vi "Checkbarcode.vi"(10 "String In":string="123456789\u0003") -> (2 "Complete":bool)   [LabVIEW 2014]
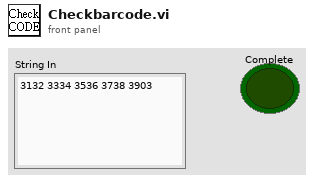
[diagram p1: front panel]
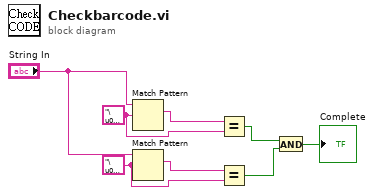
[diagram p0: block diagram]
diagram:
  w6 = "\u0003" ("regular expression")
  w1 = "\u0002" ("regular expression")
  n1 = Match Pattern(string="String In", regular expression=w1) -> (match substring=w8:string)  [unwired: 1 in, 3 out]
  n2 = Match Pattern(string="String In", regular expression=w6) -> (match substring=w7:string)  [unwired: 1 in, 3 out]
  n3 = Equal?(x=w8, y=w1) -> (x = y?=w5:bool)
  n4 = Equal?(x=w7, y=w6) -> (x = y?=w4:bool)
  n5 = And(x=w5, y=w4) -> (x .and. y?=→"Complete":bool)
